vi "Radau5_Build Error.vi"(11 "error code":i32) -> (0 "error out":errorcluster)   [LabVIEW 2017, in "NI_DAE.lvlib"]
uses:
  <vilib>/gmath/NI_DAE.lvlib
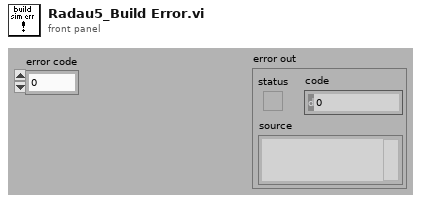
[diagram p1: front panel]
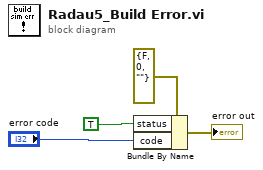
[diagram p0: block diagram]
diagram:
  n1 = Bundle By Name(cluster=errorcluster {"status"=FALSE, "code"=0, "source"=""} ("error"), "status"=TRUE ("error.status"), "code"="error code") -> (→"error out":errorcluster)
